vi "test_kpi_panel.vi"() -> ()   [LabVIEW 2024]
uses:
  FlexCompute_grpc_client/RPC Messages/rfcontrol_KPIData.ctl
  FlexCompute_grpc_client/RPC Messages/rfcontrol_Status.ctl
  FlexCompute_grpc_client/RPC Messages/rfcontrol_Empty.ctl
  FlexCompute_grpc_client/FlexCompute_grpc_client.lvlib
panel:
  out "error out":errorcluster
  out "Response Data":T1
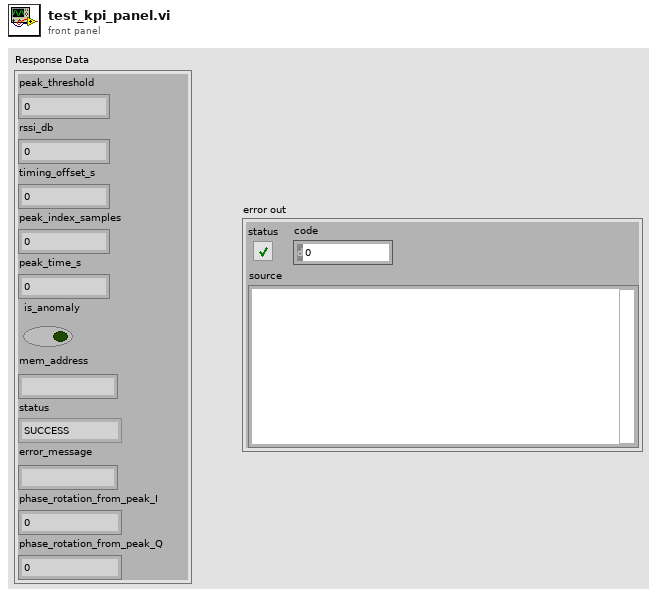
[diagram p1: front panel]
types:
  T1 = typedef "FlexCompute_grpc_client.lvlib/rfcontrol_KPIData.ctl" = cluster{"peak_threshold":dbl, "rssi_db":dbl, "timing_offset_s":dbl, "peak_index_samples":i32, "peak_time_s":dbl, "is_anomaly":bool, "mem_address":string, "status":T2, "error_message":string, "phase_rotation_from_peak_I":sgl, "phase_rotation_from_peak_Q":sgl}
  T2 = typedef "FlexCompute_grpc_client.lvlib/rfcontrol_Status.ctl" = enum32{"SUCCESS", "ERROR"}
  T3 = typedef "FlexCompute_grpc_client.lvlib/rfcontrol_Empty.ctl" = cluster{"void":string}
  T4 = typedef "grpc-lvsupport-release.lvlib/grpcId.ctl" = u64
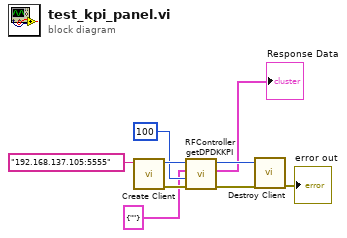
[diagram p0: block diagram]
diagram:
  n1 = call "Create Client.vi"("address"="192.168.137.105:5555") -> ("error out"=w9:errorcluster, "gRPC ID Out"=w8:T4)  [unwired: 9 in]
  n2 = call "RFController getDPDKKPI.vi"("error in"=w9, "timeout (ms)"=100, "Request Data"=T3 {"void"=""}, "gRPC ID"=w8) -> ("error out"=w7:errorcluster, "Response Data"=→"Response Data":T1, "gRPC ID out"=w6:T4)  [unwired: 5 in]
  n3 = call "Destroy Client.vi"("error in"=w7, "gRPC ID"=w6) -> ("error out"=→"error out":errorcluster)  [unwired: 9 in]
